vi "Write Motor Obj.vi"(8 "error in (no error)":errorcluster, 10 "Hardware.lvlib:Motor.lvlib:Motor.lvclass":refnum<class "Motor.lvclass">, 11 "Motor Configuration in":refnum<class "Motor Configuration.lvclass">) -> (0 "error out":errorcluster, 3 "Motor Configuration out":refnum<class "Motor Configuration.lvclass">)   [LabVIEW 2016, in "Hardware.lvlib" / "Motor.lvlib" / "Motor Configuration.lvclass"]
uses:
  <userlib>/Common Components/Hardware/Motor/Motor Config/Motor Configuration.lvclass
  <userlib>/Common Components/Hardware/Motor/Motor/Motor.lvclass
  <userlib>/Common Components/Hardware/Motor/Motor Config/Motor Configuration.lvclass/Motor Configuration.ctl
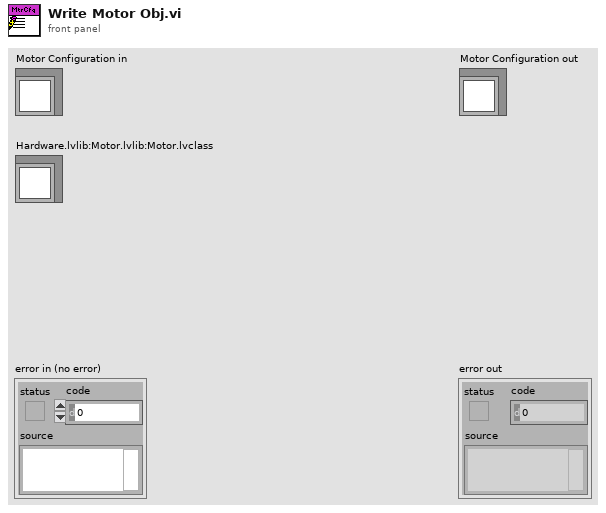
[diagram p1: front panel]
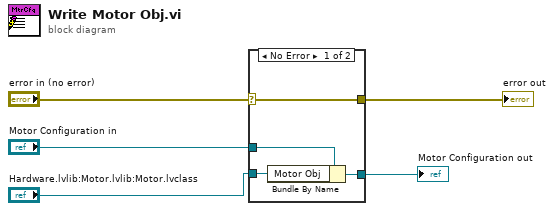
[diagram p0: block diagram]
diagram:
  n1 = case shown="No Error" "error in (no error)" {
    selector: "error in (no error)" -> [w6 w11]
    tunnel: [w9 w10] -> w5
    tunnel: "Motor Configuration in" -> [w8 w10]
    tunnel: "Hardware.lvlib:Motor.lvlib:Motor.lvclass" -> [w7 _]
    tunnel: [w6 w11] -> w1
    frame No Error {
      n2 = Bundle By Name(cluster=w8, "Motor Obj"=w7) -> (w9:refnum<class "Motor Configuration.lvclass">)
    }
    frame Error {
    }
  }
  "error out" <- w1
  "Motor Configuration out" <- w5
